vi "myRIO_BRig_RT_TCP__v3__PortC.vi"(0 "input_hTCP":refnum<k5>, 1 "input_AI1":i16, 2 "input_AI0":i16, 3 "input_I_connected_TCP":bool, 5 "input_iBlock":u16, 7 "input_spout":enum16{"Left", "Right"}(ring), 9 "input_iTrial":u16, 11 "input_error":errorcluster, 12 "input_countTrial":u16, 13 "input_iState":T1) -> (4 "output_hTCP":refnum<k5>, 14 "output_countTrial":u16, 15 "output_error":errorcluster)   [LabVIEW 2014]
uses:
  myRIO_BRig_RT__Case_Exp_stateList.ctl
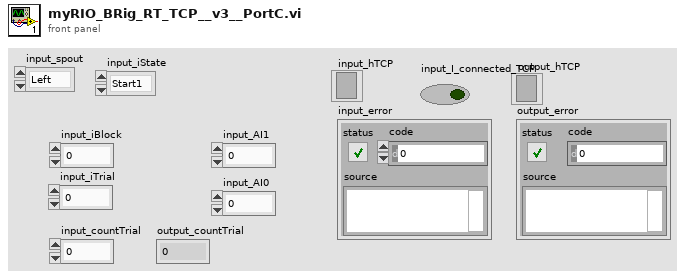
[diagram p1: front panel]
types:
  T1 = typedef "myRIO_BRig_RT__Case_Exp_stateList.ctl" = enum16{"Start1", "Start2", "Start3", "saveSettings1", "saveSettings2", "saveSettings3", "saveSettings4", "saveSettings_LC_ENL_l1", "saveSettings_LC_ENL_l2", "saveSettings_LC_Cue_l1", "saveSettings_LC_Cue_l2", "saveSettings6_LC_l1_Other", "SaveSettings6_LC_l2_Other", "setSettings_Audio", "setSettings_Laser", "initBlock_pre", "initBlock", "initBlock2", "initBlock_post", "initTrial_pre", "initTrial", "initTrial2", "initTrial3", "initTrial4", "initTrial_LC_ENL1", "initTrial_LC_Cue1", "initTrial_LC_Cue1_2", "initTrial_LC_Sel", "initTrial_post", "ENL1_pre", "ENL1", "ENL1_post", "ENL1Penalty_pre", "ENL1Penalty", "ENL2_pre", "ENL2", "ENL2Penalty_pre", "ENL2Penalty", "Cue1_pre", "Cue1", "Cue1_post", "Cue1Penalty_pre", "Cue1Penalty", "Cue2_pre", "Cue2", "Cue2Penalty_pre", "Cue2Penalty", "Selection_pre", "Selection", "Select_post", "SelectReward_pre", "SelectReward", "SelectRewardPost_pre", "SelectRewardPost", "SelectWrong_pre", "SelectWrong", "SelectWrong_post", "SelectTimeout_pre", "SelectTimeout", "SelectTimeout_post", "endTrial_pre", "endTrial1", "endTrial2", "endTrial3", "endTrial_post", "endBlock_pre", "endBlock", "endBlock_post", "endExp", "commConnect", "commUpload_pre", "commUpload_dataBlock", "commUpload_dataCurrent", "commUpload_dataExp", "commUpload_dataLC", "commUpload_dataTrial", "commUpload_post", "saveData_pre", "saveData_dataBlock", "saveData_dataCurrent", "saveData_dataExp", "saveData_dataLC", "saveData_dataTrial", "saveData_post", "empty_endBlock1", "empty_endBlock2", "empty_endTrial1", "empty_endTrial2", "empty_endTrial3", "empty_endTrial4", "empty_endTrial5", "dummyState", "dummyState_endBlock"}
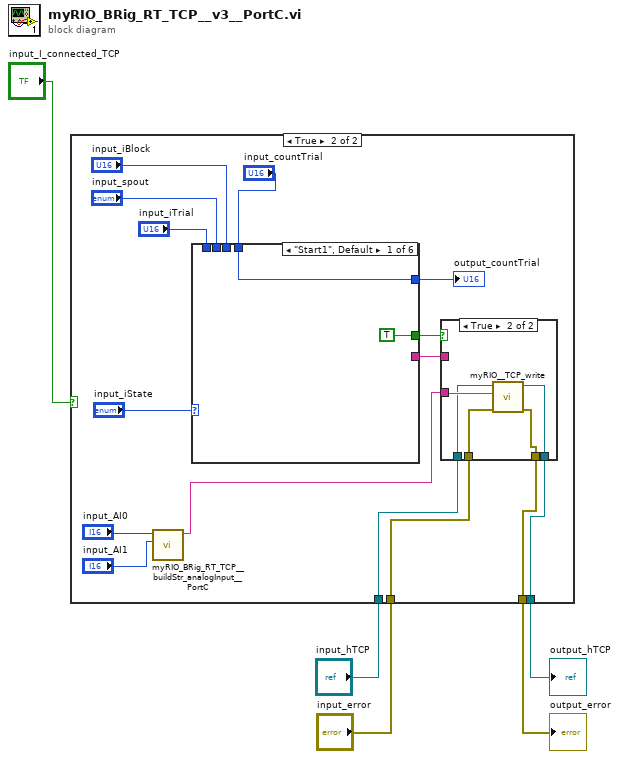
[diagram p0: block diagram]
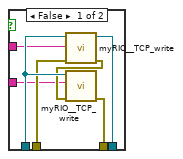
[diagram p3: hidden frame]
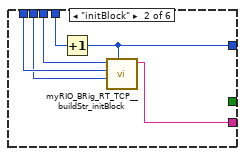
[diagram p4: hidden frame]
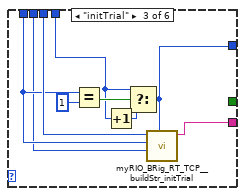
[diagram p5: hidden frame]
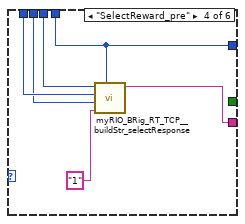
[diagram p6: hidden frame]
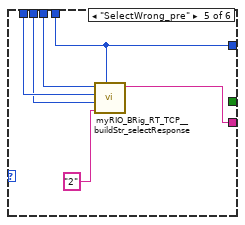
[diagram p7: hidden frame]
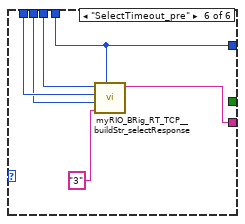
[diagram p8: hidden frame]
diagram:
  n1 = case shown="True" "input_I_connected_TCP" {
    tunnel: "input_hTCP" -> [w6 w16]
    tunnel: "input_error" -> [w7 w15]
    tunnel: [w7 w14] -> w2
    tunnel: [w6 w13] -> w1
    frame False {
    }
    frame True {
      n2 = call "myRIO_BRig_RT_TCP__buildStr_analogInput__PortC.vi"("input_AI1"="input_AI1", "input_AI0"="input_AI0") -> ("output_str_analogInput"=w10:string)  [unwired: 9 in]
      n3 = case shown="\"Start1\", Default" "input_iState" {
        tunnel: "input_iTrial" -> [_ w38 w44 w56 w63 w69]
        tunnel: "input_spout" -> [_ w37 w43 w55 w62 w68]
        tunnel: "input_iBlock" -> [_ w40 w45 w57 w61 w67]
        tunnel: [_ w39 w46 w53 w59 w65] -> w17
        tunnel: [TRUE _ _ _ _ _] -> w18
        tunnel: "input_countTrial" -> [w35 w42 w48 w54 w60 w66]
        tunnel: [w35 w41 w47 w54 w60 w66] -> w8
        frame "Start1", Default {
        }
        frame "initBlock" {
          n4 = Increment(x=w42) -> (x+1=w41:u16)
          n5 = call "myRIO_BRig_RT_TCP__buildStr_initBlock.vi"("input_countTrial"=w41, "input_spout"=w37, "input_iTrial"=w38, "input_iBlock"=w40) -> ("output_str_initBlock"=w39:string)  [unwired: 7 in]
        }
        frame "initTrial" {
          n6 = Equal?(x=w44, y=u16 1) -> (x = y?=w50:bool)
          n7 = Increment(x=w48) -> (x+1=w49:u16)
          n8 = Select(t=w48, s=w50, f=w49) -> (s? t:f=w47:u16)
          n9 = call "myRIO_BRig_RT_TCP__buildStr_initTrial.vi"("input_countTrial"=w47, "input_spout"=w43, "input_iTrial"=w44, "input_iBlock"=w45) -> ("output_str_initTrial"=w46:string)  [unwired: 7 in]
        }
        frame "SelectReward_pre" {
          n10 = call "myRIO_BRig_RT_TCP__buildStr_selectResponse.vi"("input_countTrial"=w54, "input_str"="1", "input_spout"=w55, "input_iTrial"=w56, "input_iBlock"=w57) -> ("output_str_selectResponse"=w53:string)  [unwired: 6 in]
        }
        frame "SelectWrong_pre" {
          n11 = call "myRIO_BRig_RT_TCP__buildStr_selectResponse.vi"("input_countTrial"=w60, "input_str"="2", "input_spout"=w62, "input_iTrial"=w63, "input_iBlock"=w61) -> ("output_str_selectResponse"=w59:string)  [unwired: 6 in]
        }
        frame "SelectTimeout_pre" {
          n12 = call "myRIO_BRig_RT_TCP__buildStr_selectResponse.vi"("input_countTrial"=w66, "input_str"="3", "input_spout"=w68, "input_iTrial"=w69, "input_iBlock"=w67) -> ("output_str_selectResponse"=w65:string)  [unwired: 6 in]
        }
      }
      "output_countTrial" <- w8
      n13 = case shown="True" w18 {
        tunnel: w17 -> [w27 _]
        tunnel: w16 -> [w29 w32]
        tunnel: w15 -> [w28 w33]
        tunnel: [w23 w31] -> w14
        tunnel: [w25 w30] -> w13
        tunnel: w10 -> [w24 w34]
        frame False {
          n14 = call "myRIO__TCP_write.vi"("input_error"=w28, "input_packet"=w27, "input_hTCP"=w29) -> ("output_error"=w26:errorcluster, "output_hTCP"=w25:refnum<k5>)  [unwired: 6 in, 1 out]
          n15 = call "myRIO__TCP_write.vi"("input_error"=w26, "input_packet"=w24, "input_hTCP"=w29) -> ("output_error"=w23:errorcluster)  [unwired: 6 in, 2 out]
        }
        frame True {
          n16 = call "myRIO__TCP_write.vi"("input_error"=w33, "input_packet"=w34, "input_hTCP"=w32) -> ("output_error"=w31:errorcluster, "output_hTCP"=w30:refnum<k5>)  [unwired: 6 in, 1 out]
        }
      }
    }
  }
  "output_hTCP" <- w1
  "output_error" <- w2
